vi "LVtime2Exceltime.vi"(1 "LabVIEW Time":timestamp) -> (0 "Time in Excel Format":dbl format="%#_10f")   [LabVIEW 2021]
doc: "transfer LabVIEW Datetime to Excel datetime.\n2015-02-04 11:03:05\n蒋松\njiangsong@outlook.com"
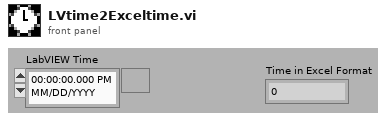
[diagram p1: front panel]
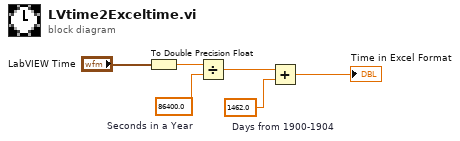
[diagram p0: block diagram]
diagram:
  w3 = 1462.0  # Days from 1900-1904
  w5 = 86400.0  # Seconds in a Year
  n1 = To Double Precision Float(number="LabVIEW Time") -> (double precision float=w6:dbl)
  n2 = Divide(x=w6, y=w5) -> (x/y=w4:dbl)
  n3 = Add(x=w4, y=w3) -> (x+y=→"Time in Excel Format":dbl)
